vi "P-541 Startup.vi"(0 "VISA Ref":refnum<visa-resource-name>, 7 "Axis Name":string, 11 "Error In":errorcluster) -> (4 "VISA Ref Out":refnum<visa-resource-name>, 15 "Error Out":errorcluster)   [LabVIEW 2020]
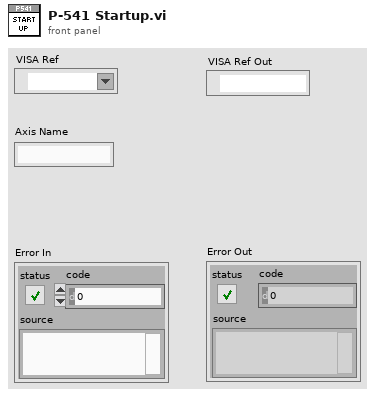
[diagram p1: front panel]
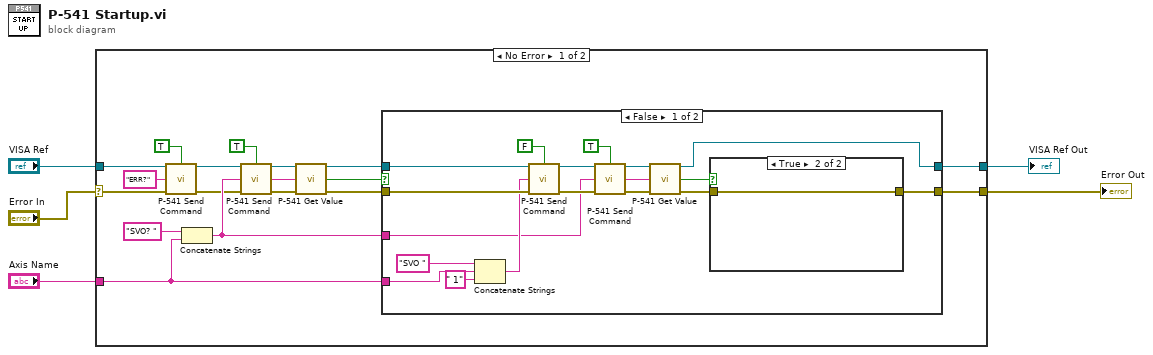
[diagram p0: block diagram]
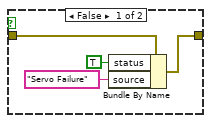
[diagram p2: hidden frame]
diagram:
  n1 = case shown="No Error" "Error In" {
    selector: "Error In" -> [w9 w49]
    tunnel: "VISA Ref" -> [w10 w50]
    tunnel: "Axis Name" -> [w15 _]
    tunnel: [w13 w50] -> w2
    tunnel: [w12 w49] -> w1
    frame No Error {
      n2 = call "P-541 Send Command.vi"("VISA Ref"=w10, "Wait for Reply (T)"=TRUE, "Command"="ERR?", "Error In"=w9) -> ("VISA Ref Dup"=w7:refnum<visa-resource-name>, "Error Out"=w8:errorcluster)  [unwired: 8 in, 2 out]
      n3 = Concatenate Strings("SVO? " ("Command"), w15) -> (w14:string)
      n4 = call "P-541 Send Command.vi"("VISA Ref"=w7, "Wait for Reply (T)"=TRUE, "Command"=w14, "Error In"=w8) -> ("VISA Ref Dup"=w21:refnum<visa-resource-name>, "Reply"=w20:string, "Error Out"=w19:errorcluster)  [unwired: 8 in, 1 out]
      n5 = call "P-541 Get Value.vi"("VISA Pass Thru"=w21, "Cmd Reply"=w20, "Error In"=w19) -> ("VISA Ref Dup"=w18:refnum<visa-resource-name>, "Bool"=w17:bool, "Error Out"=w16:errorcluster)  [unwired: 9 in, 1 out]
      n6 = case shown="False" w17 {
        tunnel: w18 -> [w40 w48]
        tunnel: w16 -> [w36 w47]
        tunnel: [w25 w48] -> w13
        tunnel: [w24 w47] -> w12
        tunnel: w15 -> [w37 _]
        tunnel: w14 -> [w28 _]
        frame False {
          n7 = Concatenate Strings("SVO " ("string"), w37, " 1" ("string")) -> (w35:string)
          n8 = call "P-541 Send Command.vi"("VISA Ref"=w40, "Wait for Reply (T)"=FALSE, "Command"=w35, "Error In"=w36) -> ("VISA Ref Dup"=w30:refnum<visa-resource-name>, "Error Out"=w29:errorcluster)  [unwired: 8 in, 2 out]
          n9 = call "P-541 Send Command.vi"("VISA Ref"=w30, "Wait for Reply (T)"=TRUE, "Command"=w28, "Error In"=w29) -> ("VISA Ref Dup"=w32:refnum<visa-resource-name>, "Reply"=w33:string, "Error Out"=w34:errorcluster)  [unwired: 8 in, 1 out]
          n10 = call "P-541 Get Value.vi"("VISA Pass Thru"=w32, "Cmd Reply"=w33, "Error In"=w34) -> ("VISA Ref Dup"=w25:refnum<visa-resource-name>, "Bool"=w27:bool, "Error Out"=w26:errorcluster)  [unwired: 9 in, 1 out]
          n11 = case shown="True" w27 {
            tunnel: w26 -> [w43 w46]
            tunnel: [w42 w46] -> w24
            frame False {
              n12 = Bundle By Name(cluster=w43, "status"=TRUE, "source"="Servo Failure") -> (w42:errorcluster)
            }
            frame True {
            }
          }
        }
        frame True {
        }
      }
    }
    frame Error {
    }
  }
  "Error Out" <- w1
  "VISA Ref Out" <- w2
